vi "IsErrorUX.vi"(8 "error in (no error)":errorcluster) -> (0 "error out":errorcluster, 3 "Is Error UX?":bool)   [LabVIEW 2019, in "LabErrorUX.lvclass"]
uses:
  LabErrorUX.lvclass
  LabErrorUX.lvclass/LabErrorUX.ctl
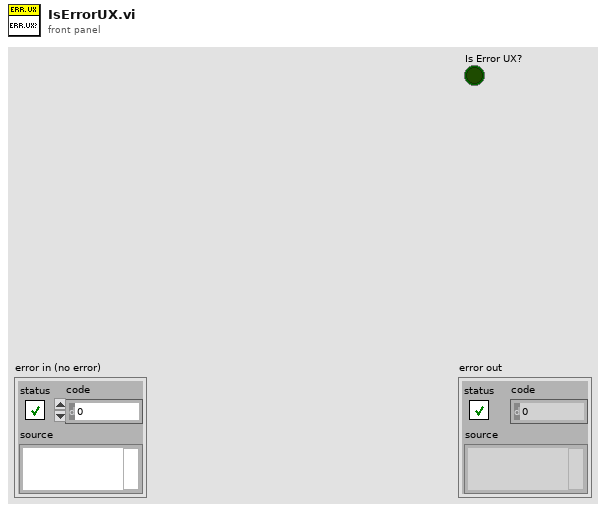
[diagram p1: front panel]
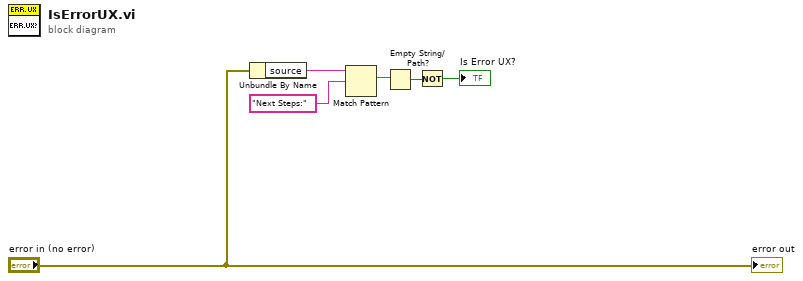
[diagram p0: block diagram]
diagram:
  n1 = Unbundle By Name("error in (no error)") -> ("source"=w5:string)
  n2 = Match Pattern(string=w5, regular expression="Next Steps:") -> (match substring=w3:string)  [unwired: 1 in, 3 out]
  n3 = Empty String/Path?(string/path=w3) -> (empty?=w2:bool)
  n4 = Not(x=w2) -> (.not. x?=→"Is Error UX?":bool)
  "error out" <- "error in (no error)"
